vi "Write_Data_Test_Json.vi"(8 "error in (no error)":errorcluster caption="entrée d'erreur (pas d'erreur)", 10 "Data Test":string, 11 "Firebase Benches P2193 en entrée":refnum<class "Firebase Benches P2193.lvclass">) -> (0 "error out":errorcluster caption="sortie d'erreur", 3 "Firebase Benches P2193 en sortie":refnum<class "Firebase Benches P2193.lvclass">)   [LabVIEW 2020, in "Library Instrument & Equipement.lvlib" / "Library FireBase.lvlib" / "Firebase Benches P2193.lvclass"]
uses:
  Firebase Benches P2193.lvclass
  Firebase Benches P2193.lvclass/Firebase Benches P2193.ctl
  JSON API/JSON Value/Set from JSON string.vi
  JSON API/JSON Value/JSON Value.lvclass
  JSON API/Variant JSON/Variant JSON.lvlib
  JSON API/Get Polymorphic/JSON GetSet.lvlib
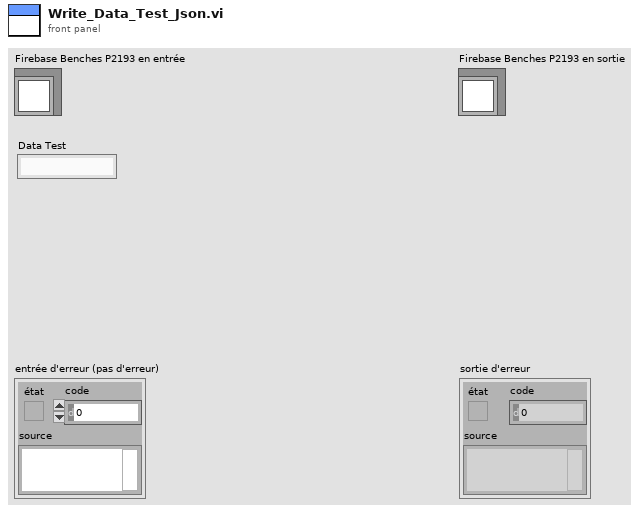
[diagram p1: front panel]
types:
  T1 = cluster{"Result":cluster{"booleanValue":bool}, "Name":cluster{"stringValue":string}, "StartOfTest":cluster{"timestampValue":string}, "EndOfTest":cluster{"timestampValue":string}, "limit":cluster{"mapValue":cluster{"fields":cluster{"Lower":cluster{"stringValue":string}, "Upper":cluster{"stringValue":string}}}}, "Value":cluster{"stringValue":string}, "Type":cluster{"stringValue":string}, "MainTest":cluster{"stringValue":string}}
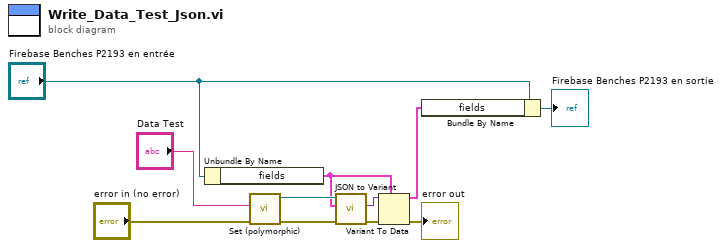
[diagram p0: block diagram]
diagram:
  n1 = Unbundle By Name("Firebase Benches P2193 en entrée") -> ("fields"=w1:T1)
  n2 = call-poly "Set (polymorphic).vi"("error in (no error)"="error in (no error)", "JSON stream"="Data Test") -> ("error out"=w9:errorcluster, "JSON Value out"=w11:refnum<class "JSON Value.lvclass">)  [unwired: 7 in, 1 out]
  n3 = call "JSON to Variant.vi"("error in (no error)"=w9, "Variant (Data Type)"=w1, "JSON Value"=w11) -> ("error out"=w10:errorcluster, "Variant out"=w8:variant)  [unwired: 7 in]
  n4 = Variant To Data(error in=w10, type=w1, Variant=w8) -> (data=w7:T1, error out=→"error out":errorcluster)
  n5 = Bundle By Name(cluster="Firebase Benches P2193 en entrée", "fields"=w7) -> (→"Firebase Benches P2193 en sortie":refnum<class "Firebase Benches P2193.lvclass">)
